vi "Create Response Headers.vi"(5 "Response Headers in":refnum<class "Response Headers.lvclass">, 8 "error in (no error)":errorcluster, 11 "Response Headers":string) -> (0 "error out":errorcluster, 3 "Response Headers out":refnum<class "Response Headers.lvclass">)   [LabVIEW 2018, in "REST Client_JKI.lvlib" / "Response Headers.lvclass"]
uses:
  Response Headers.lvclass
  Response Headers.lvclass/Response Headers.ctl
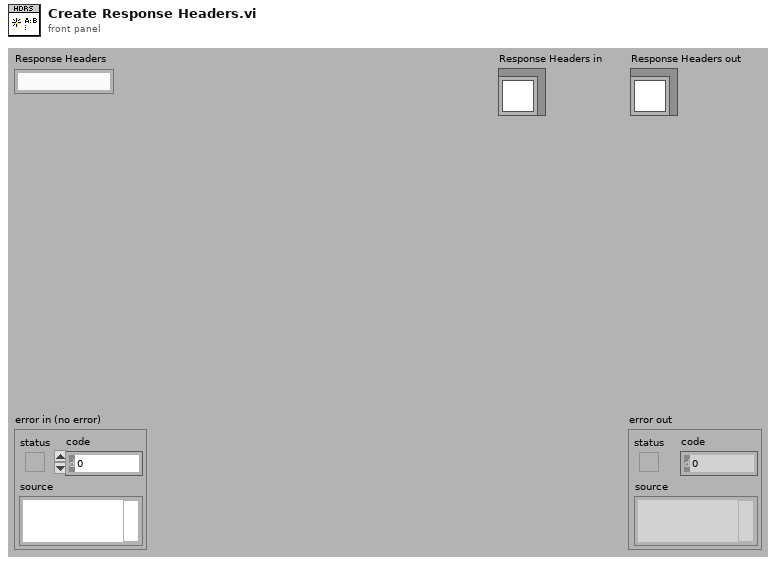
[diagram p1: front panel]
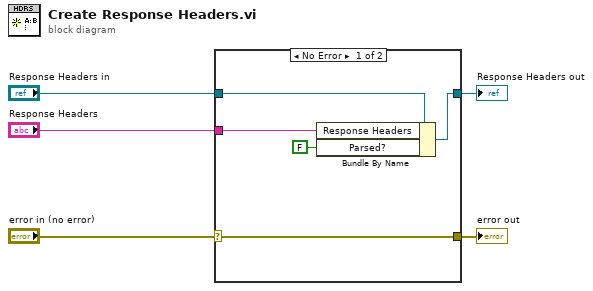
[diagram p0: block diagram]
diagram:
  n1 = case shown="No Error" "error in (no error)" {
    selector: "error in (no error)" -> [w7 w12]
    tunnel: [w7 w12] -> w4
    tunnel: [w9 w11] -> w2
    tunnel: "Response Headers in" -> [w10 w11]
    tunnel: "Response Headers" -> [w8 _]
    frame No Error {
      n2 = Bundle By Name(cluster=w10, "Response Headers"=w8, "Parsed?"=FALSE) -> (w9:refnum<class "Response Headers.lvclass">)
    }
    frame Error {
    }
  }
  "error out" <- w4
  "Response Headers out" <- w2
